vi "syringepump_standalone.vi"() -> ()   [LabVIEW 2020]
panel:
  in  "Set rate":dbl format="%#_4g"
  in  "dia (mm)":dbl=0.1 caption="Dia (mm)" min=0.1 max=50.0
  in  "Serial Port":refnum<visa-resource-name>="COM4"
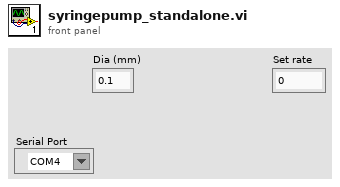
[diagram p1: front panel]
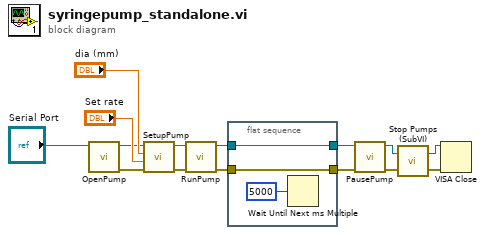
[diagram p0: block diagram]
diagram:
  n1 = call "OpenPump.vi"("VISA Refnum in"="Serial Port") -> ("error out"=w11:errorcluster, "VISA Refnum out"=w12:refnum<visa-resource-name>)  [unwired: 9 in]
  n2 = call "SetupPump.vi"("error in (no error)"=w11, "Set rate"="Set rate", "dia (mm)"="dia (mm)", "VISA Refnum in"=w12) -> ("error out"=w2:errorcluster, "VISA Refnum out"=w1:refnum<visa-resource-name>)  [unwired: 5 in, 1 out]
  n3 = call "RunPump.vi"("error in (no error)"=w2, "VISA Refnum in"=w1) -> ("error out"=w8:errorcluster, "VISA Refnum out"=w10:refnum<visa-resource-name>)  [unwired: 8 in]
  n4 = flat-sequence {
    tunnel: w10 -> [w18]
    tunnel: [w18] -> w9
    tunnel: w8 -> [w17]
    tunnel: [w17] -> w7
    frame #0 {
      n5 = Wait Until Next ms Multiple(millisecond multiple=u32 5000) -> ()  [unwired: 1 out]
    }
  }
  n6 = call "PausePump.vi"("error in (no error)"=w7, "VISA Refnum in"=w9) -> ("error out"=w3:errorcluster, "VISA Refnum out"=w4:refnum<visa-resource-name>)  [unwired: 8 in]
  n7 = call "Stop Pumps (SubVI).vi"("error out 2"=w3, "VISA resource name out 2"=w4) -> ("error out"=w5:errorcluster, "VISA resource name out"=w6:refnum<visa-resource-name>)
  n8 = VISA Close(VISA resource name=w6, error in (no error)=w5) -> ()  [unwired: 1 out]
